vi "Vol-Play.vi"(6 "State":T1, 7 "Cycle number (in)":i32, 8 "error in (no error)":errorcluster, 10 "Stop button pressed":bool, 11 "Number of Frames":u32) -> (0 "error out":errorcluster, 1 "Cycle number (out)":i32, 2 "Speed data waveform graph":dbl[](graph), 3 "I mage ref out":T2, 4 "Playback stopped":bool)   [LabVIEW 2017]
uses:
  <vilib>/vision/Image Controls.llb/IMAQ Image.ctl
  Timelapse Viewer/Typedefs/Speed Viewer States enum.ctl
  Timelapse Viewer/Typedefs/Select Play-Stop button to show.ctl
  Timelapse Viewer/Globals/gl_Time series viewer globals.vi
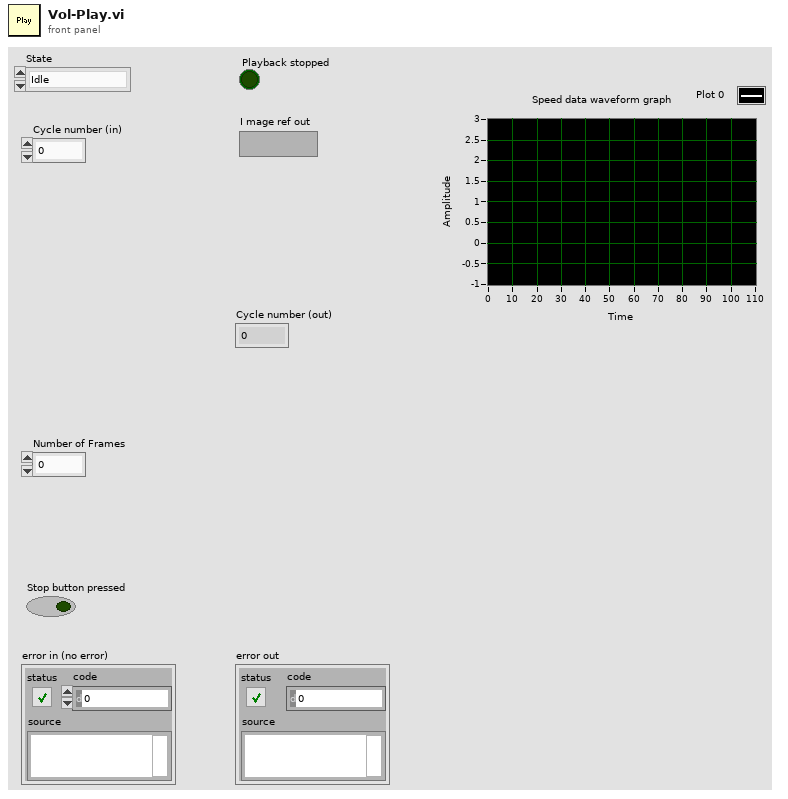
[diagram p1: front panel]
types:
  T1 = typedef "Speed Viewer States enum.ctl" = enum16{"Idle", "Initialise", "Playback", "Scroll bar event", "Speed cursor event", "Back to start", "Exit"}
  T2 = typedef "IMAQ Image.ctl" = refnum<image>
  T3 = typedef "Time series viewer refs.ctl" = cluster{"This VI":refnum<vi>, "Image control":refnum<vi>, "AVI Mode ind":refnum<vi>, "Play":refnum<vi>, "Stop":refnum<vi>, "Back":refnum<vi>, "Scrollbar":refnum<vi>, "Video length info":refnum<vi>, "Expected speed values":refnum<vi>, "Intensity":refnum<vi>, "Path":refnum<vi>, "Selection sliders":refnum<vi>, "Speed Graph ref":refnum<vi>, "Frame rate set (fps)":refnum<vi>, "Channel to load":refnum<vi>, "Number of rows to generate":refnum<vi>, "Colour":refnum<vi>}
  T4 = typedef "Select Play-Stop button to show.ctl" = enum16{"Show Play button", "Show Stop button"}
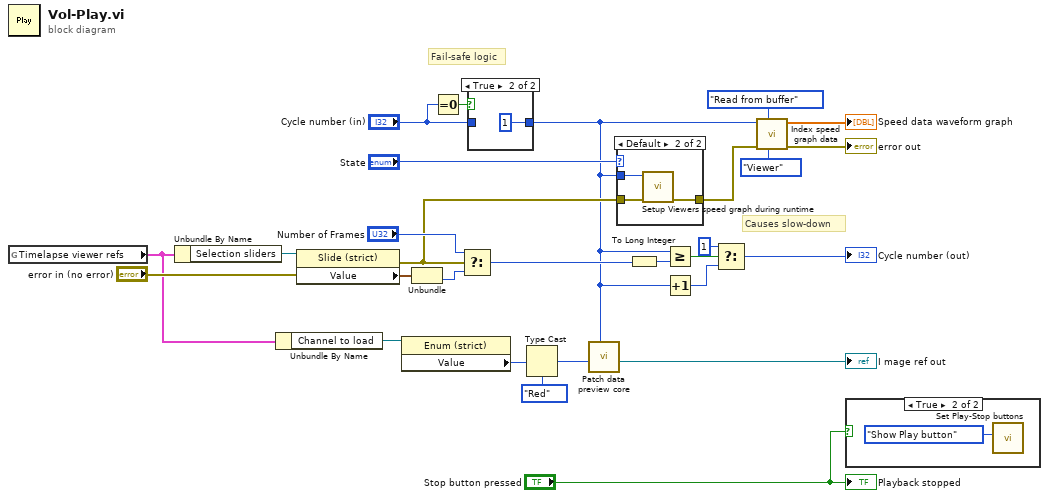
[diagram p0: block diagram]
diagram:
  # "Causes slow-down"
  # "Fail-safe logic"
  n1 = global read "gl_Time series viewer globals.vi" "Timelapse viewer refs"() -> (w10:T3)
  n2 = Unbundle By Name(w10) -> ("Selection sliders"=w21:refnum<vi>)
  n3 = Unbundle By Name(w10) -> ("Channel to load"=w9:refnum<vi>)
  n4 = property class="Slide (strict)"(reference=w21, error in="error in (no error)") -> (error out=w13:errorcluster, "Value"=w20:cluster{i32, i32})  [unwired: 1 out]
  n5 = property class="Enum (strict)"(reference=w9) -> ("Value"=w4:enum16{"Show red channel", "Show green channel"})  [unwired: 1 in, 2 out]
  n6 = Unbundle(w20) -> (w19:i32)  [unwired: 1 out]
  n7 = Equal To 0?(x="Cycle number (in)") -> (x = 0?=w7:bool)
  n8 = Select(t="Number of Frames", s=w13, f=w19) -> (s? t:f=w18:u32)
  n9 = case shown="True" w7 {
    tunnel: [w29 1 ("Value")] -> w5
    tunnel: "Cycle number (in)" -> [w29 _]
    frame False {
    }
    frame True {
    }
  }
  n10 = Type Cast(type=enum16{"Red", "Green"}."Red" ("Channel to load"), x=w4) -> (*(type *) &x=w3:enum16{"Red", "Green"})
  n11 = call "Patch data preview core.vi"("Global cycle number among all trials"=w5, "Channel to load"=w3) -> ("Image ref (montage)"=→"I mage ref out":T2)  [unwired: 8 in, 1 out]
  n12 = case shown="Default" "State" {
    tunnel: w13 -> [w31 w34]
    tunnel: [w31 w33] -> w12
    tunnel: w5 -> [_ w32]
    frame "Speed cursor event" {
    }
    frame Default {
      n13 = call "Setup Viewers speed graph during runtime.vi"("error in (no error)"=w34, "Frame number or cycle number"=w32) -> ("error out"=w33:errorcluster)  [unwired: 9 in]
    }
  }
  n14 = To Long Integer(number=w18) -> (32bit integer=w23:i32)
  n15 = Greater Or Equal?(x=w5, y=w23) -> (x >= y?=w27:bool)
  n16 = Increment(x=w5) -> (x+1=w28:i32)
  n17 = Select(t=1, s=w27, f=w28) -> (s? t:f=→"Cycle number (out)":i32)
  n18 = call "Index speed graph data.vi"("Caller"=enum16{"Viewer", "Exporter"}."Viewer", "Buffer operation (read from internal buffer)"=enum16{"Update buffer", "Read from buffer"}."Read from buffer", "error in (no error)"=w12, "Gobal frame number in Timelapse data/master video (1 based)"=w5) -> ("error out"=→"error out":errorcluster, "Speed data waveform graph"=→"Speed data waveform graph":dbl[])  [unwired: 5 in, 1 out]
  n19 = case shown="True" "Stop button pressed" {
    frame False {
    }
    frame True {
      n20 = call "Set Play-Stop buttons.vi"("Function"=Select_Play-Stop_button_to_show."Show Play button") -> ()  [unwired: 10 in, 1 out]
    }
  }
  "Playback stopped" <- "Stop button pressed"
